vi "Pre Iterate.vi"(8 "error in (no error)":errorcluster, 11 "Example Actor in":refnum<class "Example Actor.lvclass">) -> (0 "error out":errorcluster, 3 "Example Actor out":refnum<class "Example Actor.lvclass">)   [LabVIEW 2023, in "Example Iterator NR Actor Auto Iteration Notification.lvlib" / "Example Actor.lvclass"]
doc: "Method called before the iterations"
uses:
  Example Actor.lvclass
  Example Actor.lvclass/Example Actor.ctl
  <userlib>/_OpenG.lib/time/time.llb/openg_time.lvlib
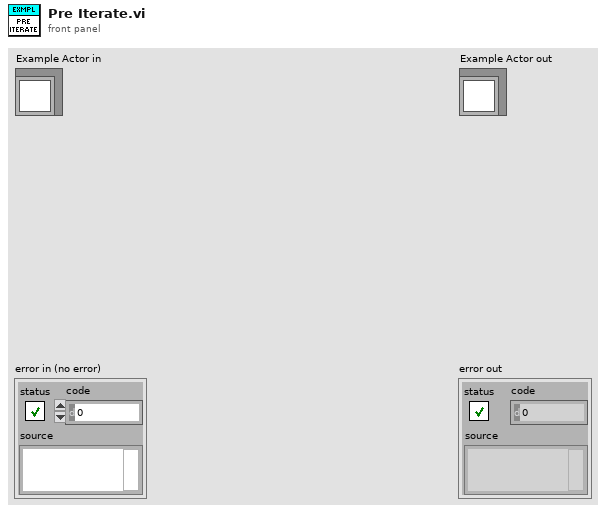
[diagram p1: front panel]
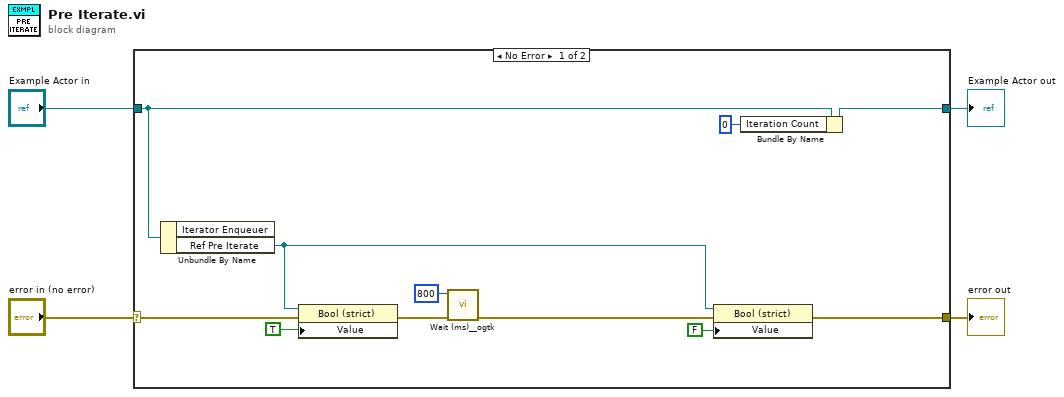
[diagram p0: block diagram]
diagram:
  n1 = case shown="No Error" "error in (no error)" {
    selector: "error in (no error)" -> [w9 w17]
    tunnel: [w5 w17] -> w3
    tunnel: [w7 w16] -> w1
    tunnel: "Example Actor in" -> [w10 w16]
    frame No Error {
      n2 = Unbundle By Name(w10) -> ("Ref Pre Iterate"=w8:refnum<vi>)  [unwired: 1 out]
      n3 = property class="Bool (strict)"(reference=w8, error in=w9, "Value"=TRUE) -> (error out=w12:errorcluster)  [unwired: 1 out]
      n4 = call <userlib>:"Wait (ms)__ogtk.vi"("error in (no error)"=w12, "milliseconds to wait"=u32 800) -> ("error out"=w11:errorcluster)  [unwired: 8 in, 1 out]
      n5 = property class="Bool (strict)"(reference=w8, error in=w11, "Value"=FALSE) -> (error out=w5:errorcluster)  [unwired: 1 out]
      n6 = Bundle By Name(cluster=w10, "Iteration Count"=0) -> (w7:refnum<class "Example Actor.lvclass">)
    }
    frame Error {
    }
  }
  "error out" <- w3
  "Example Actor out" <- w1
